vi "Action Engine Test.vi"() -> ()   [LabVIEW 2021]
uses:
  Controls/Timer Actions.ctl
panel:
  out "Clock Output":bool
  out "Time Elapsed":dbl
  in  "Stop Button":bool
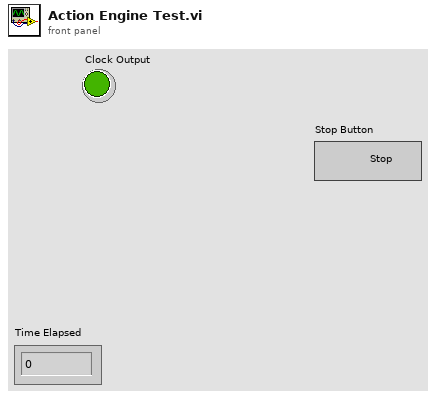
[diagram p1: front panel]
types:
  T1 = typedef "Timer Actions.ctl" = enum16{"Start Timer", "Restart Timer", "Check Timer", "Pause Timer", "Reset Timer", "Exit Timer"}
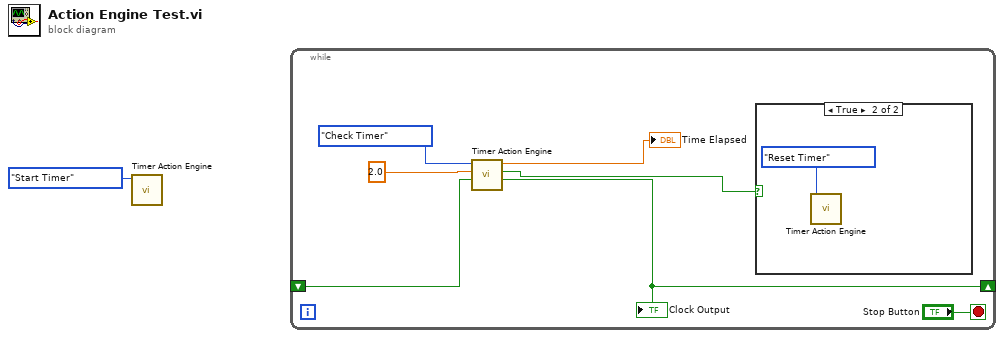
[diagram p0: block diagram]
diagram:
  n1 = call "Timer Action Engine.vi"("Action"=Timer_Actions."Start Timer") -> ()  [unwired: 7 in, 4 out]
  n2 = while {
    shift-right: [w3] -> _
    shift-left: _ -> [w2]
    stop <- "Stop Button" stop-if-true
    n3 = call "Timer Action Engine.vi"("Current State"=w2, "Time Duration (s)"=2.0, "Action"=Timer_Actions."Check Timer") -> ("Clock Output"=w3:bool, "Pulse Out"=w5:bool, "Time Elapsed"=→"Time Elapsed":dbl)  [unwired: 5 in, 1 out]
    "Clock Output" <- w3
    n4 = case shown="True" w5 {
      frame False {
      }
      frame True {
        n5 = call "Timer Action Engine.vi"("Action"=Timer_Actions."Reset Timer") -> ()  [unwired: 7 in, 4 out]
      }
    }
  }
